vi "Read Value (Variant).vi"(7 "field name":string, 8 "error in (no error)":errorcluster, 10 "value":variant, 11 "Value in":refnum<class "Value.lvclass">) -> (0 "error out":errorcluster, 2 "value out":variant, 3 "Value out":refnum<class "Value.lvclass">)   [LabVIEW 2020, in "Value.lvlib" / "Value.lvclass"]
uses:
  Value.lvclass
  <vilib>/ErrorRing/Error Ring.xnode
  3e63842f-1b42-44b7-bfbc-53574ae558bd.vi
  0df52538-0c37-4fc1-a2a6-aa64d23bd73e.vi
  ea7cb730-9445-4e63-a674-7488b051f0a2.vi
  ecc6d044-d1d6-4258-b554-93b542f000c4.vi
  f0dd0353-13dc-4229-be36-72f5216b3ba3.vi
  663b7534-5be4-4c26-8693-775dffd107bf.vi
  6d95b702-a3d4-47fa-b99c-6e9c691d9abd.vi
  334379f0-c2c1-4fd4-b37a-a75153a3c3c1.vi
  22215a59-2fe5-468e-8a76-07a567f1422d.vi
  3b673ad6-c2bb-415d-ac32-dac8d0585a62.vi
  4907590c-51dd-452d-854a-3f23d6337043.vi
  91e94b60-106e-4a8f-bb72-5d9817169e6a.vi
  c7390ac7-e1e0-4f30-b90a-9159575d946d.vi
  aaf6655d-cd8e-45f8-b77e-a22837ed21e0.vi
  830d96f2-0dcb-4e12-99cb-9e6dde05f73e.vi
  77dc8c9c-6059-4e17-8748-14fb7ec0ac2f.vi
  a9875d30-4bd9-4a8c-a52c-f68dec12aa6b.vi
  6dbc08b8-92b8-4054-99f1-d97896c52856.vi
  c55a9e90-05cb-4a8a-8098-6274f5663967.vi
  316c9c8d-b543-4ebf-942d-59175514938d.vi
  229b0493-3b28-4ef3-8240-f1556a969e00.vi
  76e9d66a-8186-463b-a0b5-702645c41f9e.vi
  c324c6c0-264f-44f1-9003-e2f03347ce10.vi
  99229403-bf4d-41b1-8e34-2119cf99b534.vi
  94649a53-8ca4-4095-9f16-4726c07ca332.vi
  d57c28cb-9096-4c65-b10b-a5dea6344eea.vi
  a983453c-48a8-483e-9635-4b6015360bbf.vi
  3184ba56-7df3-4453-b731-c59013ebea68.vi
  6054442b-7a6b-42bc-83b9-383781339b04.vi
  6affac03-527b-4ec4-b0fc-9a513264455a.vi
  a9131e02-a07e-4dd8-b605-98a98183cd4d.vi
  df721e5c-d840-4c3d-88a1-754951405b27.vi
  37bd5290-b6b7-48eb-a0fa-e2d498b26fe2.vi
  1f354738-e960-4e7d-8bfb-2b975031cf57.vi
  eb45627c-0224-4171-a2ca-7d038fcf7cb5.vi
  763b9c78-21ee-42ab-85a7-a612ad3e0854.vi
  b475763c-3eeb-44d5-9789-6e92f77c8c05.vi
  7e13b756-e5dd-4f30-8145-3e48ab5751a0.vi
  311b836b-25cf-44d6-867a-da423852ab29.vi
  884a57a7-1cc5-4241-a283-3421418f3c32.vi
  e5b34253-12a8-4f36-ae48-ef8a9a19dc9f.vi
  9a6462e7-f1a7-4896-b94c-43e163632ccd.vi
  919939b4-f74b-49d6-a078-a721f5adc92b.vi
  7b5734c8-9551-4087-a43c-2e9c6be36d77.vi
  e7c0ed72-c8d2-4a6e-8d95-57b650344be6.vi
  78a636ab-c8c7-43d5-9c2f-ed25fd418a22.vi
  3f976d8e-f489-4d6c-8102-c644feb36fb3.vi
  2b071918-53f3-414b-a359-069b1376627a.vi
  19a97183-6244-455f-abdd-dba3394d2b07.vi
  <vilib>/Utility/error.llb/Error Cluster From Error Code.vi
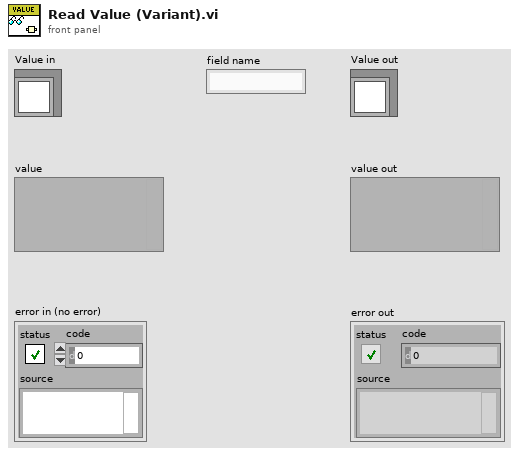
[diagram p1: front panel]
types:
  T1 = typedef "Value.lvlib/Type Code.ctl" = enum8{"Null", "Bool", "BoolA", "Int8", "Int8A", "Int16", "Int16A", "Int32", "Int32A", "Int64", "Int64A", "UInt8", "UInt8A", "UInt16", "UInt16A", "UInt32", "UInt32A", "UInt64", "UInt64A", "Float32", "Float32A", "Float64", "Float64A", "String", "StringA", "Struct", "StructA", "Union", "UnionA", "Any", "AnyA"}
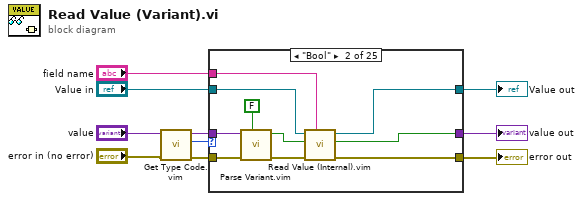
[diagram p0: block diagram]
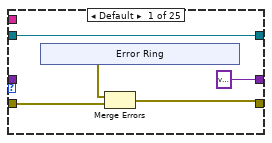
[diagram p2: hidden frame]
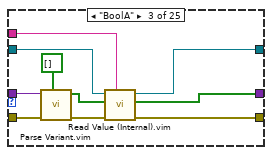
[diagram p3: hidden frame]
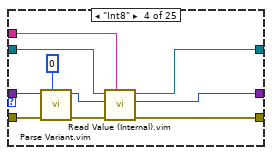
[diagram p4: hidden frame]
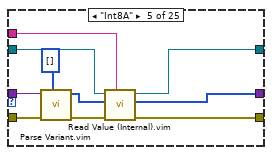
[diagram p5: hidden frame]
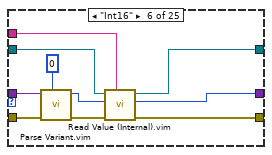
[diagram p6: hidden frame]
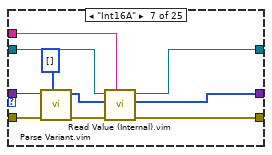
[diagram p7: hidden frame]
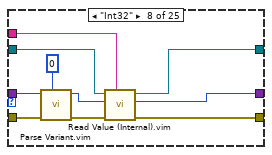
[diagram p8: hidden frame]
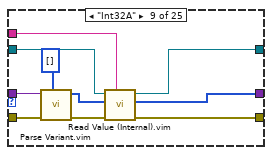
[diagram p9: hidden frame]
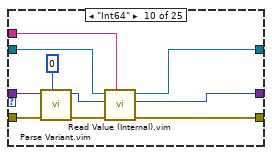
[diagram p10: hidden frame]
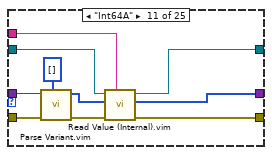
[diagram p11: hidden frame]
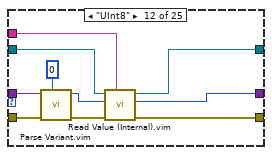
[diagram p12: hidden frame]
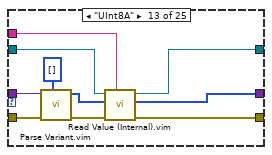
[diagram p13: hidden frame]
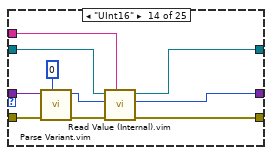
[diagram p14: hidden frame]
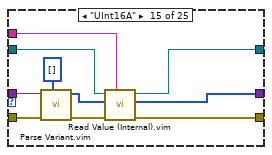
[diagram p15: hidden frame]
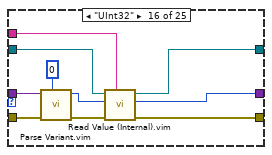
[diagram p16: hidden frame]
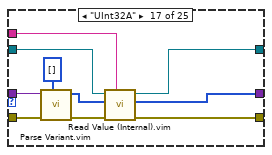
[diagram p17: hidden frame]
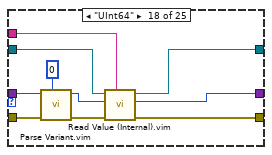
[diagram p18: hidden frame]
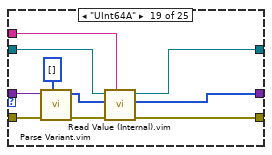
[diagram p19: hidden frame]
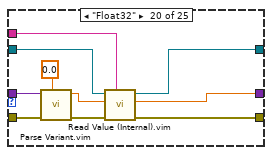
[diagram p20: hidden frame]
diagram:
  n1 = call "Get Type Code.vim"("error in"="error in (no error)", "default"="value") -> ("error out"=w8:errorcluster, "type code"=w7:T1, "value"=w6:variant)  [unwired: 7 in]
  n2 = case shown="\"Bool\"" w7 {
    tunnel: [w14 w26 w37 w47 w57 w67 w77 w87 w97 w107 w118 w127 w137 w147 w157 w167 w177 w187 w197 w207 w217 w227 w237 w247 w257] -> w4
    tunnel: w8 -> [w15 w29 w39 w49 w59 w69 w79 w89 w99 w109 w119 w129 w139 w149 w159 w169 w179 w189 w199 w209 w219 w229 w239 w249 w259]
    tunnel: [w11 w24 w35 w46 w55 w65 w75 w85 w95 w105 w116 w125 w135 w146 w155 w165 w176 w185 w195 w205 w215 w225 w235 w245 w255] -> w2
    tunnel: w6 -> [_ w23 w34 w45 w54 w64 w74 w84 w94 w104 w115 w124 w134 w145 w154 w164 w175 w184 w194 w204 w214 w224 w234 w244 w254]
    tunnel: [variant w22 w32 w43 w52 w62 w72 w82 w92 w102 w113 w122 w132 w143 w152 w162 w173 w182 w192 w202 w212 w222 w232 w242 w252] -> w5
    tunnel: "Value in" -> [w11 w21 w31 w42 w51 w61 w71 w81 w91 w101 w111 w121 w131 w142 w151 w161 w172 w181 w191 w201 w211 w221 w231 w241 w251]
    tunnel: "field name" -> [_ w20 w30 w40 w50 w60 w70 w80 w90 w100 w110 w120 w130 w140 w150 w160 w170 w180 w190 w200 w210 w220 w230 w240 w250]
    frame Default {
      n3 = xnode "Error Ring"() -> ("error out"=w13:errorcluster)
      n4 = Merge Errors(w13, w15) -> (w14:errorcluster)
    }
    frame "Bool" {
      n5 = call "Parse Variant.vim"("default"=FALSE, "error in (no error)"=w29, "value"=w23) -> ("error out"=w27:errorcluster, "value out"=w25:bool)  [unwired: 7 in]
      n6 = call "Read Value (Internal).vim"("field name"=w20, "error in"=w27, "default"=w25, "Value in"=w21) -> ("error out"=w26:errorcluster, "value"=w22:bool, "Value out"=w24:refnum<class "Value.lvclass">)  [unwired: 5 in]
    }
    frame "BoolA" {
      n7 = call "Parse Variant.vim"("default"=bool[] [], "error in (no error)"=w39, "value"=w34) -> ("error out"=w38:errorcluster, "value out"=w36:bool[])  [unwired: 7 in]
      n8 = call "Read Value (Internal).vim"("field name"=w30, "error in"=w38, "default"=w36, "Value in"=w31) -> ("error out"=w37:errorcluster, "value"=w32:bool[], "Value out"=w35:refnum<class "Value.lvclass">)  [unwired: 5 in]
    }
    frame "Int8" {
      n9 = call "Parse Variant.vim"("default"=i8 0, "error in (no error)"=w49, "value"=w45) -> ("error out"=w48:errorcluster, "value out"=w41:i8)  [unwired: 7 in]
      n10 = call "Read Value (Internal).vim"("field name"=w40, "error in"=w48, "default"=w41, "Value in"=w42) -> ("error out"=w47:errorcluster, "value"=w43:i8, "Value out"=w46:refnum<class "Value.lvclass">)  [unwired: 5 in]
    }
    frame "Int8A" {
      n11 = call "Parse Variant.vim"("default"=i8[] [], "error in (no error)"=w59, "value"=w54) -> ("error out"=w58:errorcluster, "value out"=w56:i8[])  [unwired: 7 in]
      n12 = call "Read Value (Internal).vim"("field name"=w50, "error in"=w58, "default"=w56, "Value in"=w51) -> ("error out"=w57:errorcluster, "value"=w52:i8[], "Value out"=w55:refnum<class "Value.lvclass">)  [unwired: 5 in]
    }
    frame "Int16" {
      n13 = call "Parse Variant.vim"("default"=i16 0, "error in (no error)"=w69, "value"=w64) -> ("error out"=w68:errorcluster, "value out"=w66:i16)  [unwired: 7 in]
      n14 = call "Read Value (Internal).vim"("field name"=w60, "error in"=w68, "default"=w66, "Value in"=w61) -> ("error out"=w67:errorcluster, "value"=w62:i16, "Value out"=w65:refnum<class "Value.lvclass">)  [unwired: 5 in]
    }
    frame "Int16A" {
      n15 = call "Parse Variant.vim"("default"=i16[] [], "error in (no error)"=w79, "value"=w74) -> ("error out"=w78:errorcluster, "value out"=w76:i16[])  [unwired: 7 in]
      n16 = call "Read Value (Internal).vim"("field name"=w70, "error in"=w78, "default"=w76, "Value in"=w71) -> ("error out"=w77:errorcluster, "value"=w72:i16[], "Value out"=w75:refnum<class "Value.lvclass">)  [unwired: 5 in]
    }
    frame "Int32" {
      n17 = call "Parse Variant.vim"("default"=0, "error in (no error)"=w89, "value"=w84) -> ("error out"=w88:errorcluster, "value out"=w86:i32)  [unwired: 7 in]
      n18 = call "Read Value (Internal).vim"("field name"=w80, "error in"=w88, "default"=w86, "Value in"=w81) -> ("error out"=w87:errorcluster, "value"=w82:i32, "Value out"=w85:refnum<class "Value.lvclass">)  [unwired: 5 in]
    }
    frame "Int32A" {
      n19 = call "Parse Variant.vim"("default"=i32[] [], "error in (no error)"=w99, "value"=w94) -> ("error out"=w98:errorcluster, "value out"=w96:i32[])  [unwired: 7 in]
      n20 = call "Read Value (Internal).vim"("field name"=w90, "error in"=w98, "default"=w96, "Value in"=w91) -> ("error out"=w97:errorcluster, "value"=w92:i32[], "Value out"=w95:refnum<class "Value.lvclass">)  [unwired: 5 in]
    }
    frame "Int64" {
      n21 = call "Parse Variant.vim"("default"=i64 0, "error in (no error)"=w109, "value"=w104) -> ("error out"=w108:errorcluster, "value out"=w106:i64)  [unwired: 7 in]
      n22 = call "Read Value (Internal).vim"("field name"=w100, "error in"=w108, "default"=w106, "Value in"=w101) -> ("error out"=w107:errorcluster, "value"=w102:i64, "Value out"=w105:refnum<class "Value.lvclass">)  [unwired: 5 in]
    }
    frame "Int64A" {
      n23 = call "Parse Variant.vim"("default"=i64[] [], "error in (no error)"=w119, "value"=w115) -> ("error out"=w112:errorcluster, "value out"=w117:i64[])  [unwired: 7 in]
      n24 = call "Read Value (Internal).vim"("field name"=w110, "error in"=w112, "default"=w117, "Value in"=w111) -> ("error out"=w118:errorcluster, "value"=w113:i64[], "Value out"=w116:refnum<class "Value.lvclass">)  [unwired: 5 in]
    }
    frame "UInt8" {
      n25 = call "Parse Variant.vim"("default"=u8 0, "error in (no error)"=w129, "value"=w124) -> ("error out"=w128:errorcluster, "value out"=w126:u8)  [unwired: 7 in]
      n26 = call "Read Value (Internal).vim"("field name"=w120, "error in"=w128, "default"=w126, "Value in"=w121) -> ("error out"=w127:errorcluster, "value"=w122:u8, "Value out"=w125:refnum<class "Value.lvclass">)  [unwired: 5 in]
    }
    frame "UInt8A" {
      n27 = call "Parse Variant.vim"("default"=u8[] [], "error in (no error)"=w139, "value"=w134) -> ("error out"=w138:errorcluster, "value out"=w136:u8[])  [unwired: 7 in]
      n28 = call "Read Value (Internal).vim"("field name"=w130, "error in"=w138, "default"=w136, "Value in"=w131) -> ("error out"=w137:errorcluster, "value"=w132:u8[], "Value out"=w135:refnum<class "Value.lvclass">)  [unwired: 5 in]
    }
    frame "UInt16" {
      n29 = call "Parse Variant.vim"("default"=u16 0, "error in (no error)"=w149, "value"=w145) -> ("error out"=w148:errorcluster, "value out"=w141:u16)  [unwired: 7 in]
      n30 = call "Read Value (Internal).vim"("field name"=w140, "error in"=w148, "default"=w141, "Value in"=w142) -> ("error out"=w147:errorcluster, "value"=w143:u16, "Value out"=w146:refnum<class "Value.lvclass">)  [unwired: 5 in]
    }
    frame "UInt16A" {
      n31 = call "Parse Variant.vim"("default"=u16[] [], "error in (no error)"=w159, "value"=w154) -> ("error out"=w158:errorcluster, "value out"=w156:u16[])  [unwired: 7 in]
      n32 = call "Read Value (Internal).vim"("field name"=w150, "error in"=w158, "default"=w156, "Value in"=w151) -> ("error out"=w157:errorcluster, "value"=w152:u16[], "Value out"=w155:refnum<class "Value.lvclass">)  [unwired: 5 in]
    }
    frame "UInt32" {
      n33 = call "Parse Variant.vim"("default"=u32 0, "error in (no error)"=w169, "value"=w164) -> ("error out"=w168:errorcluster, "value out"=w166:u32)  [unwired: 7 in]
      n34 = call "Read Value (Internal).vim"("field name"=w160, "error in"=w168, "default"=w166, "Value in"=w161) -> ("error out"=w167:errorcluster, "value"=w162:u32, "Value out"=w165:refnum<class "Value.lvclass">)  [unwired: 5 in]
    }
    frame "UInt32A" {
      n35 = call "Parse Variant.vim"("default"=u32[] [], "error in (no error)"=w179, "value"=w175) -> ("error out"=w178:errorcluster, "value out"=w171:u32[])  [unwired: 7 in]
      n36 = call "Read Value (Internal).vim"("field name"=w170, "error in"=w178, "default"=w171, "Value in"=w172) -> ("error out"=w177:errorcluster, "value"=w173:u32[], "Value out"=w176:refnum<class "Value.lvclass">)  [unwired: 5 in]
    }
    frame "UInt64" {
      n37 = call "Parse Variant.vim"("default"=u64 0, "error in (no error)"=w189, "value"=w184) -> ("error out"=w188:errorcluster, "value out"=w186:u64)  [unwired: 7 in]
      n38 = call "Read Value (Internal).vim"("field name"=w180, "error in"=w188, "default"=w186, "Value in"=w181) -> ("error out"=w187:errorcluster, "value"=w182:u64, "Value out"=w185:refnum<class "Value.lvclass">)  [unwired: 5 in]
    }
    frame "UInt64A" {
      n39 = call "Parse Variant.vim"("default"=u64[] [], "error in (no error)"=w199, "value"=w194) -> ("error out"=w198:errorcluster, "value out"=w196:u64[])  [unwired: 7 in]
      n40 = call "Read Value (Internal).vim"("field name"=w190, "error in"=w198, "default"=w196, "Value in"=w191) -> ("error out"=w197:errorcluster, "value"=w192:u64[], "Value out"=w195:refnum<class "Value.lvclass">)  [unwired: 5 in]
    }
    frame "Float32" {
      n41 = call "Parse Variant.vim"("default"=sgl 0.0, "error in (no error)"=w209, "value"=w204) -> ("error out"=w208:errorcluster, "value out"=w206:sgl)  [unwired: 7 in]
      n42 = call "Read Value (Internal).vim"("field name"=w200, "error in"=w208, "default"=w206, "Value in"=w201) -> ("error out"=w207:errorcluster, "value"=w202:sgl, "Value out"=w205:refnum<class "Value.lvclass">)  [unwired: 5 in]
    }
    frame "Float64" {
      n43 = call "Parse Variant.vim"("default"=0.0, "error in (no error)"=w219, "value"=w214) -> ("error out"=w218:errorcluster, "value out"=w216:dbl)  [unwired: 7 in]
      n44 = call "Read Value (Internal).vim"("field name"=w210, "error in"=w218, "default"=w216, "Value in"=w211) -> ("error out"=w217:errorcluster, "value"=w212:dbl, "Value out"=w215:refnum<class "Value.lvclass">)  [unwired: 5 in]
    }
    frame "Float32A" {
      n45 = call "Parse Variant.vim"("default"=sgl[] [], "error in (no error)"=w229, "value"=w224) -> ("error out"=w228:errorcluster, "value out"=w226:sgl[])  [unwired: 7 in]
      n46 = call "Read Value (Internal).vim"("field name"=w220, "error in"=w228, "default"=w226, "Value in"=w221) -> ("error out"=w227:errorcluster, "value"=w222:sgl[], "Value out"=w225:refnum<class "Value.lvclass">)  [unwired: 5 in]
    }
    frame "Float64A" {
      n47 = call "Parse Variant.vim"("default"=dbl[] [], "error in (no error)"=w239, "value"=w234) -> ("error out"=w238:errorcluster, "value out"=w236:dbl[])  [unwired: 7 in]
      n48 = call "Read Value (Internal).vim"("field name"=w230, "error in"=w238, "default"=w236, "Value in"=w231) -> ("error out"=w237:errorcluster, "value"=w232:dbl[], "Value out"=w235:refnum<class "Value.lvclass">)  [unwired: 5 in]
    }
    frame "String" {
      n49 = call "Parse Variant.vim"("default"="", "error in (no error)"=w249, "value"=w244) -> ("error out"=w248:errorcluster, "value out"=w246:string)  [unwired: 7 in]
      n50 = call "Read Value (Internal).vim"("field name"=w240, "error in"=w248, "default"=w246, "Value in"=w241) -> ("error out"=w247:errorcluster, "value"=w242:string, "Value out"=w245:refnum<class "Value.lvclass">)  [unwired: 5 in]
    }
    frame "StringA" {
      n51 = call "Parse Variant.vim"("default"=string[] [], "error in (no error)"=w259, "value"=w254) -> ("error out"=w258:errorcluster, "value out"=w256:string[])  [unwired: 7 in]
      n52 = call "Read Value (Internal).vim"("field name"=w250, "error in"=w258, "default"=w256, "Value in"=w251) -> ("error out"=w257:errorcluster, "value"=w252:string[], "Value out"=w255:refnum<class "Value.lvclass">)  [unwired: 5 in]
    }
  }
  "value out" <- w5
  "error out" <- w4
  "Value out" <- w2
